vi "AMS Gas v2.0.vi"() -> ()   [LabVIEW 2015]
uses:
  Controls/FP Sample Container.ctl
  Controls/Valve Vertical.ctl
  Controls/Valve Custom.ctl
  Controls/Freezer.ctl
  Controls/Scroll ONOFF.ctl
  Controls/Sample Transfer State Enumerator.ctl
  Controls/Sample Push State Enumerator.ctl
  Controls/Vacuum State Enumerator.ctl
  Controls/FP Control Refs Cluster.ctl
  Controls/Liquid N Valve Ref Cluster.ctl
  Controls/Main Line Valve Ref Cluster.ctl
  Controls/Sample Valve Refs.ctl
  Controls/Syringe Ctrl Refs.ctl
  Controls/AMS Gas State Enumerator.ctl
  AMS Gas/AMS Gas.lvclass
  <vilib>/ActorFramework/Message Enqueuer/Message Enqueuer.lvclass/Message Enqueuer.ctl
  Controls/Sample Line State Enumerator.ctl
  Controls/Sample Transfer Control Enumerator.ctl
  Controls/Sample Push Control Enumerator.ctl
  <vilib>/ActorFramework/Message Enqueuer/Enqueue.vi
  <vilib>/ActorFramework/Message Priority Queue/Priority Enqueue.vi
  AMS Gas Messages/Open Log Msg/Open Log Msg.lvclass
  AMS Gas Messages/Open Thermocouples Msg/Open Thermocouples Msg.lvclass
  <vilib>/ActorFramework/Stop Msg/Stop Msg.lvclass
panel:
  out "Syringe TC 2":dbl(slide)
  out "Sample Transfer State":T1
  out "Sample Push Progress Slide":u8(slide) scale=0.0..100.0
  in  "Syringe TC Graph":bool
  out "Sample Push State":T2
  out "Syringe TC":dbl(slide) scale=-200.0..50.0
  in  "Open Log":bool
  in  "Blank Button":bool
  out "Vacuum State":T3=enum."Unknown"
  out "Baratron 1":dbl(knob) scale=0.0005..1000.0
  in  "Vacuum Derivative":dbl(slide) scale=-0.01..0.01
  in  "Cylinder Home":bool
  in  "Syringe Blower":bool
  in  "Syringe Freeze":bool
  in  "Syringe Heater":bool
  in  "Piston Heater":bool
  in  "Syringe Valve":bool
  in  "Capillary Valve":bool
  in  "Syringe Container":bool
  out "Sample Transfer Progress Slide":u8(slide) scale=0.0..100.0
  in  "Cylinder Setpoint":dbl=2.6 min=0.0 max=10.0 step=0.01 format="%_3f bar"
  in  "He Line Valve DV318":bool
  in  "Push Time (sec)":dbl=inf
  out "cRIO CPU":u8(slide) scale=0.0..100.0
  out "Capillary Container":bool
  in  "Monkey Mode":bool
  out "error out":errorcluster
  in  "Scroll ON/OFF":T4
  in  "Turbo ON":bool
  out "Turbo Speed":dbl(knob) scale=0.0..100.0
  in  "Turbo Valve DV313":bool
  in  "Turbo Line Container":T5
  in  "GV400":T6
  in  "GV401":T6
  out "FV Gauge":dbl
  out "Log":string
  in  "Liquid N Master Valve HV 107":bool
  in  "Cold Bath Syringe HV 106":bool
  in  "Cold Bath Storage 1 HV 102":T7
  in  "Cold Bath Storage 2 HV 103":T7
  in  "Cold Bath Storage 3 HV 104":bool
  in  "Cold Bath Storage 4 HV 105":bool
  in  "Tank Blower 4":bool
  in  "Tank Blower 3":bool
  in  "Tank Blower 2":bool
  in  "Tank Blower 1":bool
  in  "Clear Charts":bool
  out "Baratrons Chart":cluster{"mean":dbl, "mean":dbl}(graph)
  out "Baratron 1":dbl(knob) scale=0.5..1000.0
  in  "Storage Valve 1":bool
  in  "Storage Valve 2":bool
  in  "Storage Valve 3":bool
  in  "Storage Valve 4":bool
  in  "Storage Valve 5":bool
  in  "Storage Valve 6":bool
  in  "Storage Valve 7":bool
  in  "Storage Valve 9":bool
  in  "Storage Valve 0":bool
  in  "Storage Valve 11":bool
  in  "Storage Valve 12":bool
  in  "Storage Valve 8":bool
  in  "Storage Container 1":T5
  in  "Storage Container 2":T5
  in  "Storage Container 3":T5
  in  "Storage Container 4":T5
  in  "Storage Container 5":T5
  in  "Storage Container 6":T5
  in  "Storage Container 7":T5
  in  "Storage Container 8":T5
  in  "Storage Container 9":T5
  in  "Storage Container 10":T5
  in  "Storage Container 11":T5
  in  "Storage Container 12":T5
  in  "Prep Line Valve 0 DV300":bool
  in  "Sample 1 DV314":bool
  in  "Sample 2 DV315":bool
  in  "Sample 3 DV316":bool
  in  "Sample 4 DV317":bool
  in  "Sample 5 DV318":bool
  in  "Sample 1":bool
  in  "Sample 2":bool
  in  "Sample 3":bool
  in  "Sample 4":bool
  in  "Sample 5":bool
  in  "Transfer Line Container":bool=TRUE
  in  "Preparation Container":bool
  in  "Cold Bath 1 Freeze":T8
  in  "Cold Bath 2 Freeze":T8
  in  "Cold Bath 3 Freeze":T8
  in  "Cold Bath 4 Freeze":T8
  in  "Cylinder Container":bool
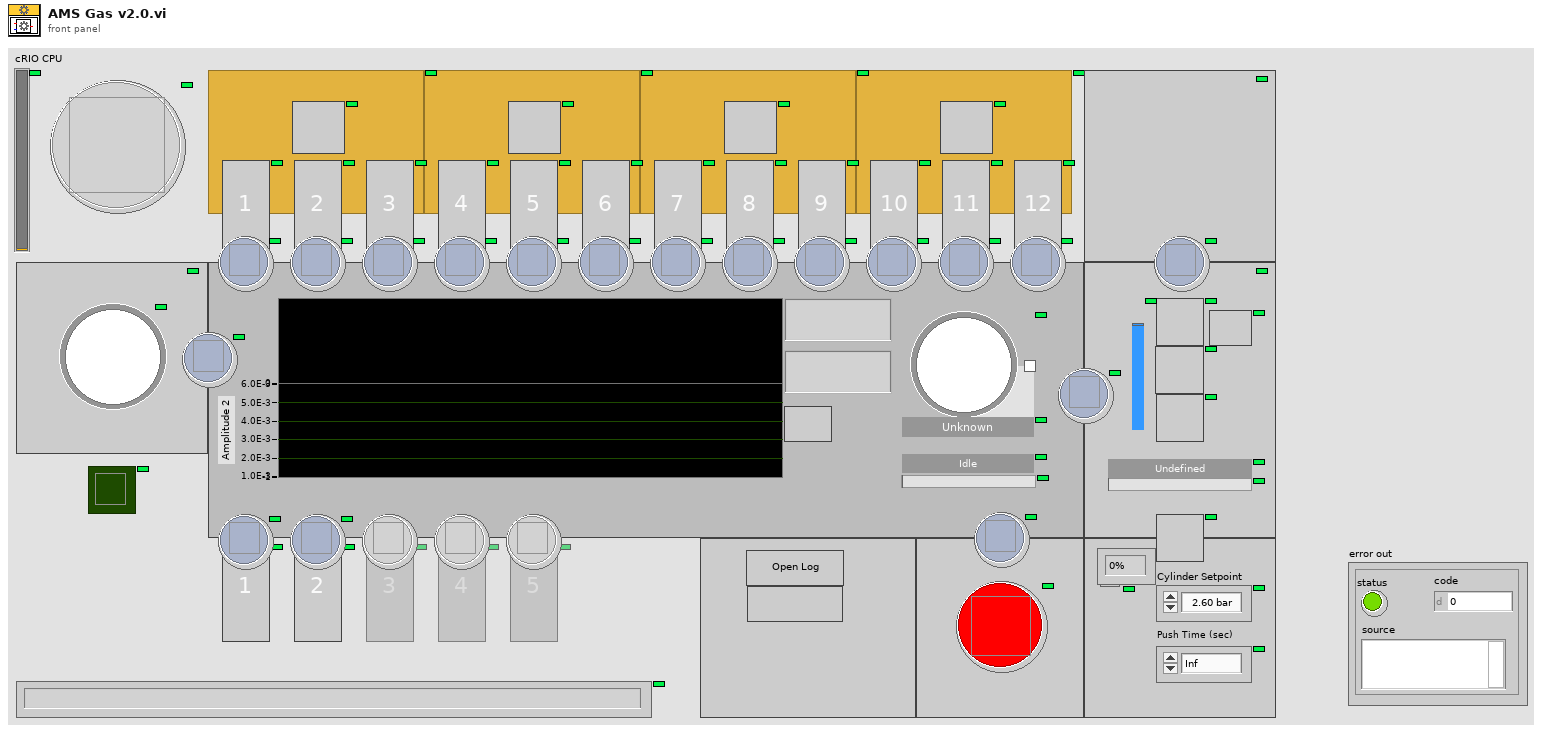
[diagram p1: front panel]
types:
  T1 = typedef "Sample Transfer State Enumerator.ctl" = enum16{"Idle", "Initialize", "Check Containers", "Check Temperatures", "Start Turbo", "Warm Up Containers", "Prepare for purging", "Purge Capillary", "Purge", "Open Containers", "Introduce Sample", "Measure Base Pressure", "Home Syringe", "Start Freezer", "Freeze Target", "Crystalize", "Initiate Stash", "Stash", "Polish", "Stop Freezers", "Push Sample", "Complete", "Abort", "Error", "Undefined"}
  T2 = typedef "Sample Push State Enumerator.ctl" = enum16{"Undefined", "Initialize", "Dilute", "Close Transfer Line", "Start Heaters", "Warm Up Syringe", "Ready to Push", "Push", "Initiate Stash", "Stash", "Complete", "Abort", "Idle", "Error"}
  T3 = typedef "Vacuum State Enumerator.ctl" = enum16{"Pressure Rising", "Plateau", "Pressure Dropping", "Valley", "Low Valley", "Leak", "Unknown"}
  T4 = typedef "Scroll ONOFF.ctl" = bool
  T5 = typedef "FP Sample Container.ctl" = bool
  T6 = typedef "Valve Vertical.ctl" = bool
  T7 = typedef "Valve Custom.ctl" = bool
  T8 = typedef "Freezer.ctl" = bool
  T9 = typedef "AMS Gas State Enumerator.ctl" = enum16{"Initialize", "Idle", "Change to Manual", "Change to Auto", "Shutdown"}
  T10 = typedef "FP Control Refs Cluster.ctl" = cluster{"Liquid N Valve References":T11, "Main Line Valve Refs":T12, "Transfer Line Container":refnum<vi>, "Storage Containers":refnum<vi>[], "Sample Refs":T13, "Syringe Ctrl Refs ":T14, "Baratrons Chart":refnum<vi>, "Capillary Container":refnum<vi>, "Preparation Container":refnum<vi>, "Monkey Mode":refnum<vi>}
  T11 = typedef "Liquid N Valve Ref Cluster.ctl" = cluster{"Cold Bath H2O HV 100":refnum<vi>, "Cold Bath Cleaning HV 101":refnum<vi>, "Cold Bath Storage 1 HV 102":refnum<vi>, "Cold Bath Storage 2 HV 103":refnum<vi>, "Cold Bath Storage 3 HV 104":refnum<vi>, "Cold Bath Storage 4 HV 105":refnum<vi>, "Cold Bath Syringe HV 106":refnum<vi>, "Liquid N Master Valve HV 107":refnum<vi>}
  T12 = typedef "Main Line Valve Ref Cluster.ctl" = cluster{"Turbo Valve DV313":refnum<vi>, "Prep Line Valve 0 DV300":refnum<vi>, "Storage Valves":refnum<vi>[]}
  T13 = typedef "Sample Valve Refs.ctl" = cluster{"Valves":cluster{"Sample 5 DV318":refnum<vi>, "Sample 4 DV317":refnum<vi>, "Sample 3 DV316":refnum<vi>, "Sample 2 DV315":refnum<vi>, "Sample 1 DV314":refnum<vi>}, "Lines":cluster{"Sample 1":refnum<vi>, "Sample 2":refnum<vi>, "Sample 3":refnum<vi>, "Sample 4":refnum<vi>, "Sample 5":refnum<vi>}}
  T14 = typedef "Syringe Ctrl Refs.ctl" = cluster{"Syringe Home":refnum<vi>, "Syringe Freeze":refnum<vi>, "Syringe TC":refnum<vi>, "Syringe Container":refnum<vi>}
  T15 = typedef "Sample Line State Enumerator.ctl" = enum16{"All lines closed", "Sample line 1.", "Sample line 2.", "Sample line 3.", "Sample line 4.", "Sample line 5.", "Out of range"}
  T16 = typedef "Sample Transfer Control Enumerator.ctl" = enum16{"Acknowledged", "Transfer", "Stash", "Abort", "Reset to Idle"}
  T17 = typedef "Sample Push Control Enumerator.ctl" = enum16{"Acknowledged", "Push", "Stash", "Abort", "Reset to Idle"}
  T18 = typedef "Sample Container.ctl" = cluster{"Sample In":refnum<k21>, "Sample Name":refnum<k21>, "Ti Cathode":refnum<k21>, "SampleQ":refnum<queue>}
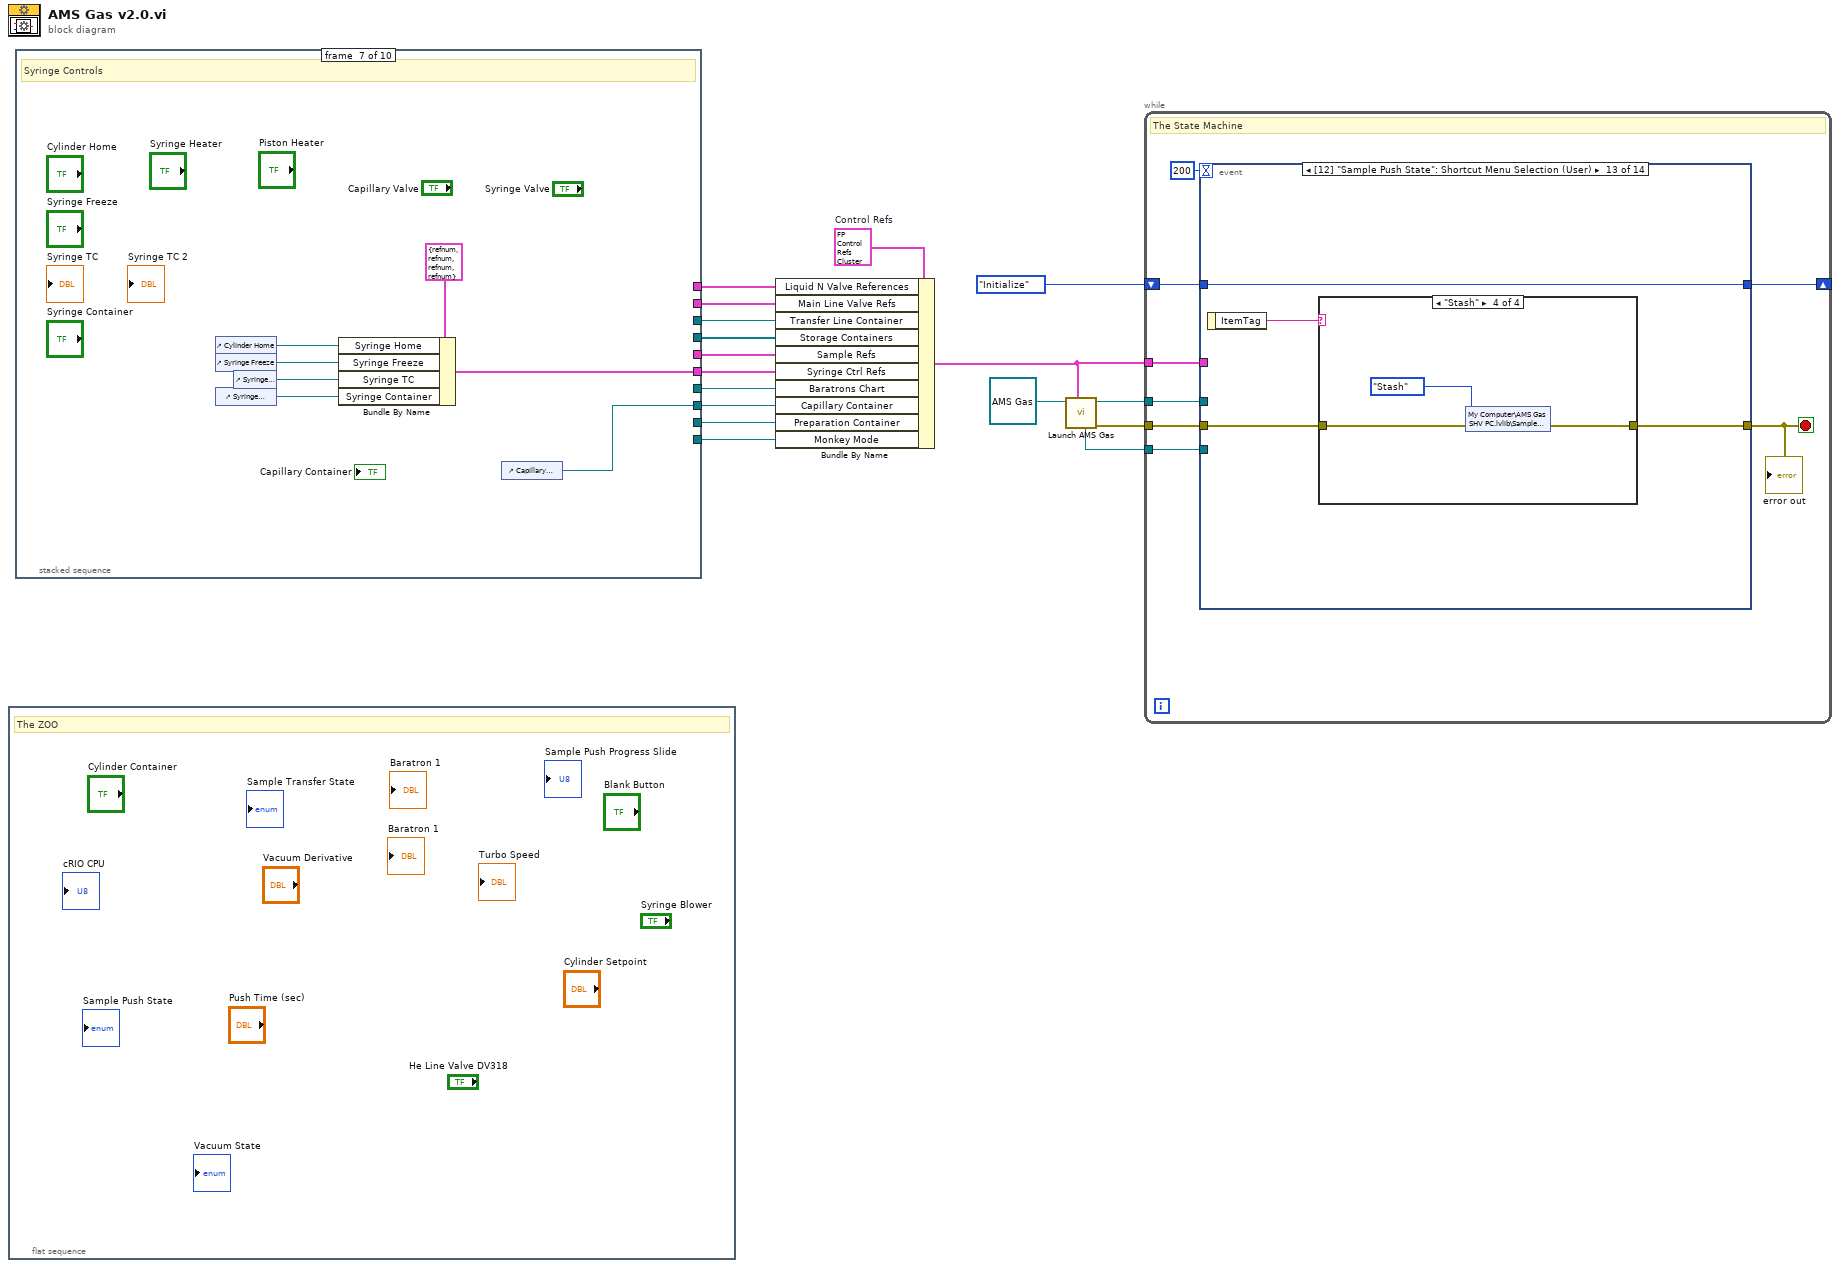
[diagram p0: block diagram]
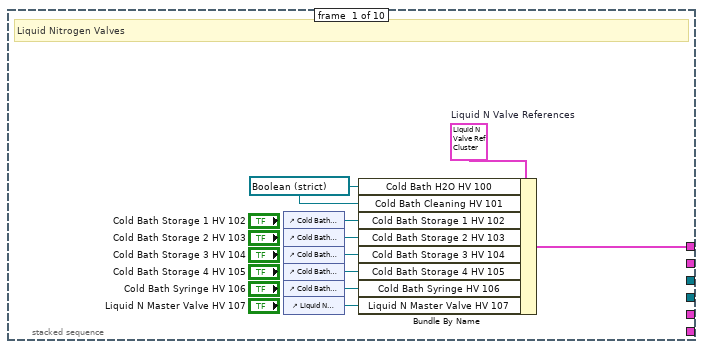
[diagram p2: hidden frame]
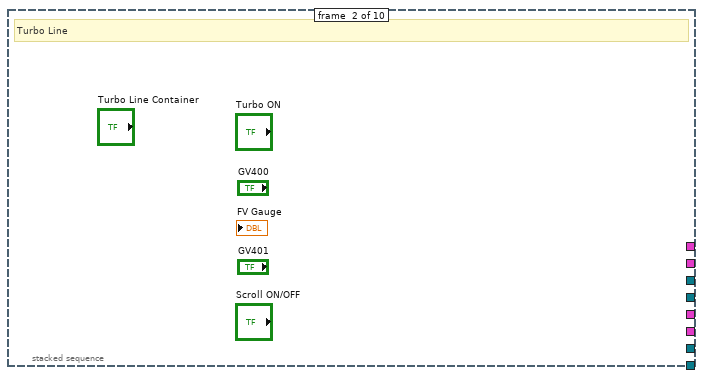
[diagram p3: hidden frame]
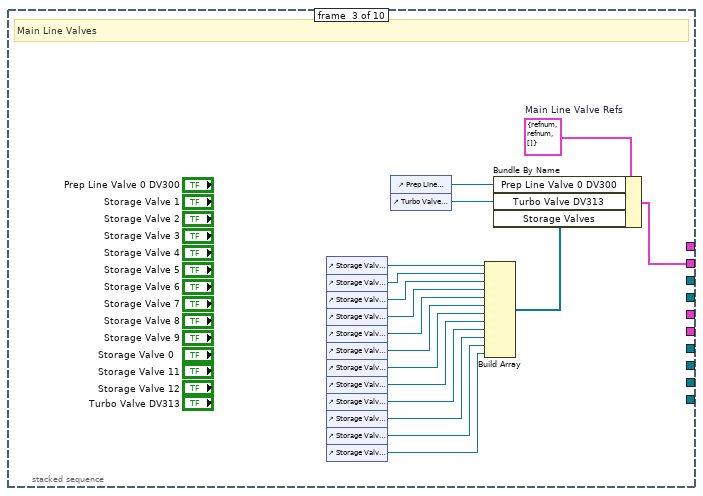
[diagram p4: hidden frame]
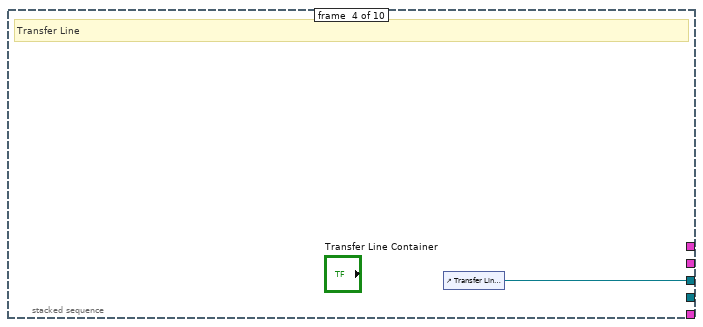
[diagram p5: hidden frame]
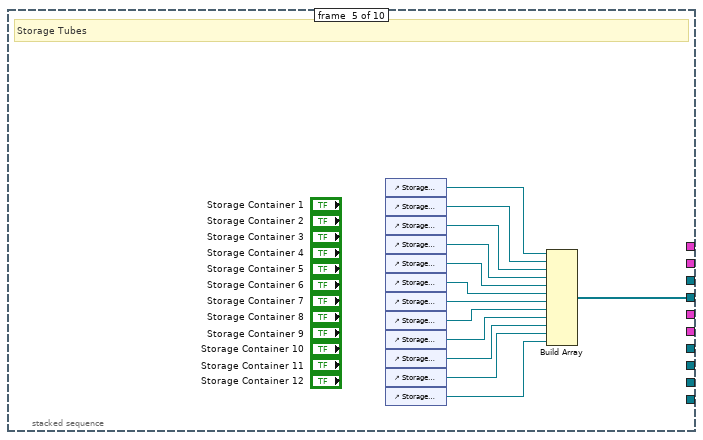
[diagram p6: hidden frame]
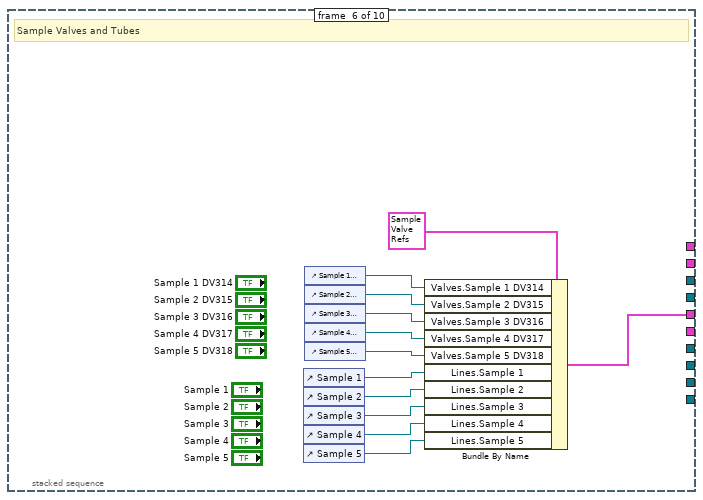
[diagram p7: hidden frame]
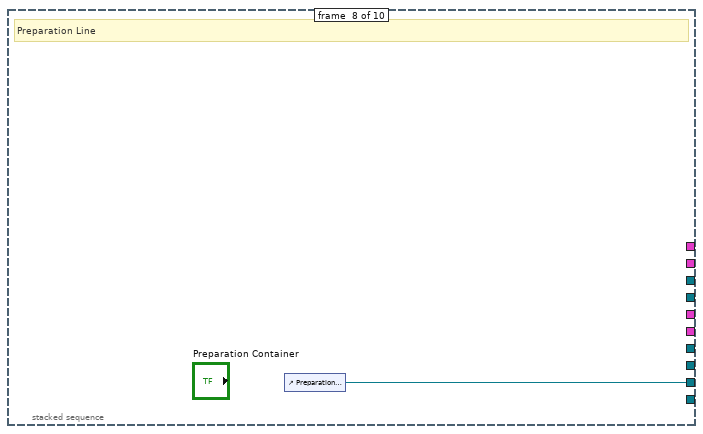
[diagram p8: hidden frame]
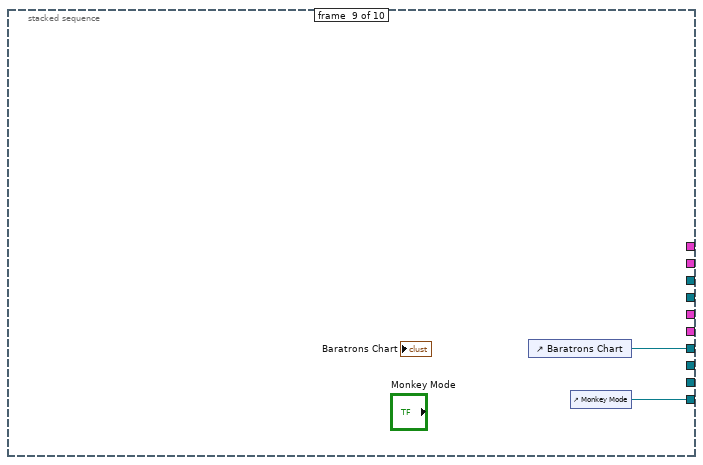
[diagram p9: hidden frame]
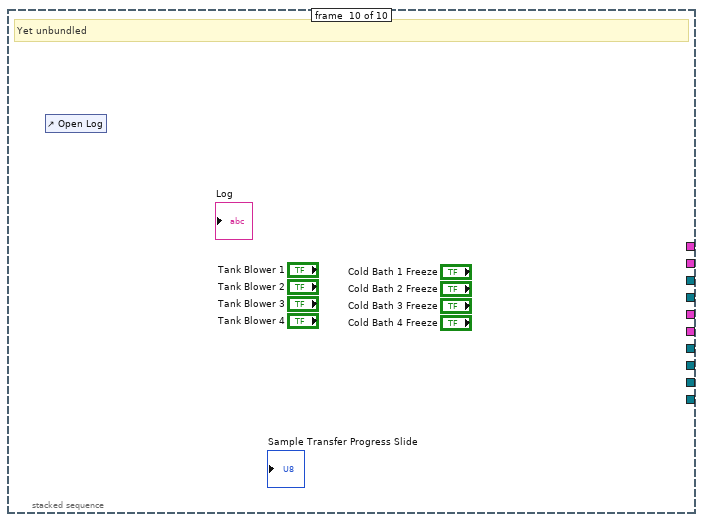
[diagram p10: hidden frame]
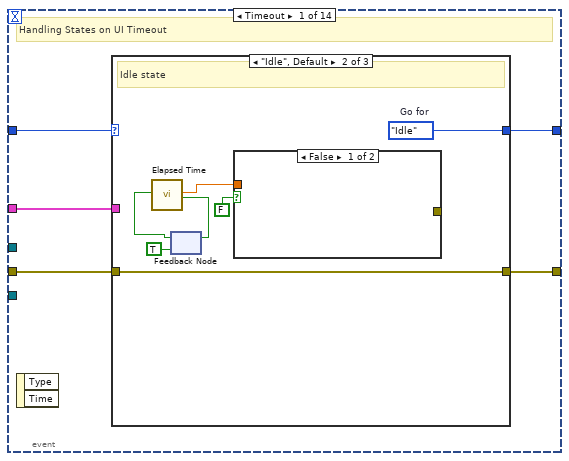
[diagram p11: hidden frame]
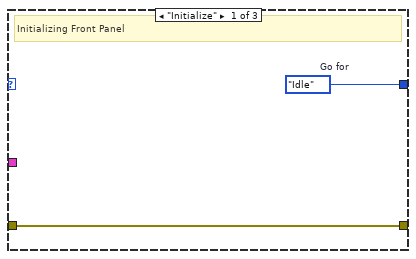
[diagram p12: hidden frame]
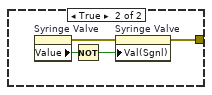
[diagram p13: hidden frame]
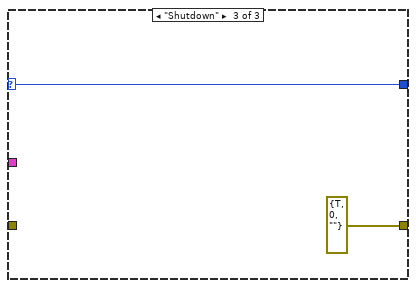
[diagram p14: hidden frame]
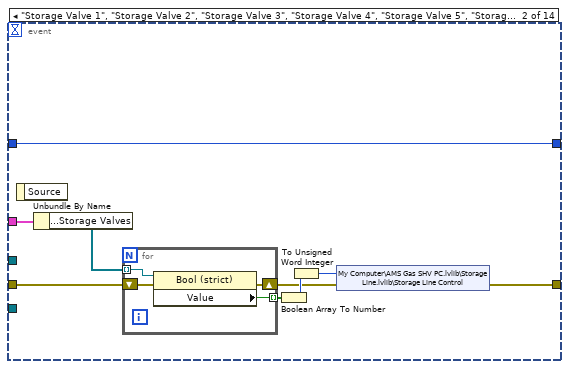
[diagram p15: hidden frame]
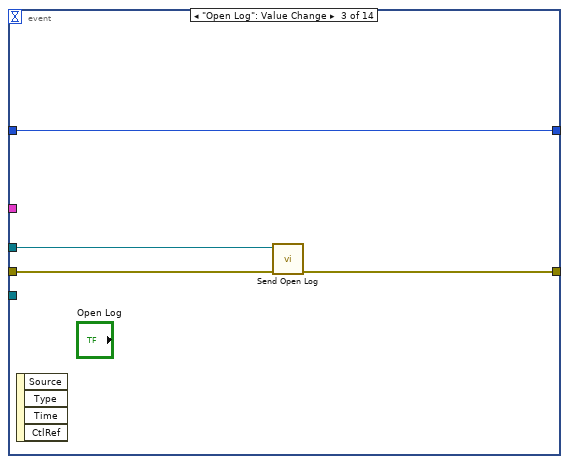
[diagram p16: hidden frame]
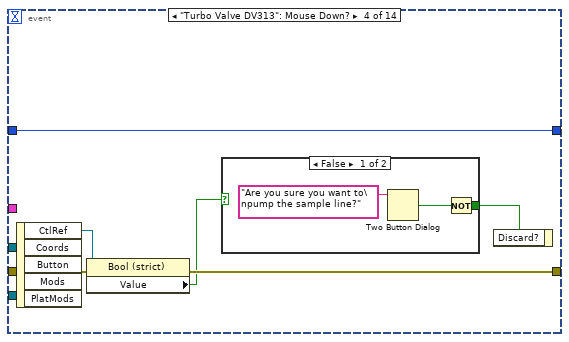
[diagram p17: hidden frame]
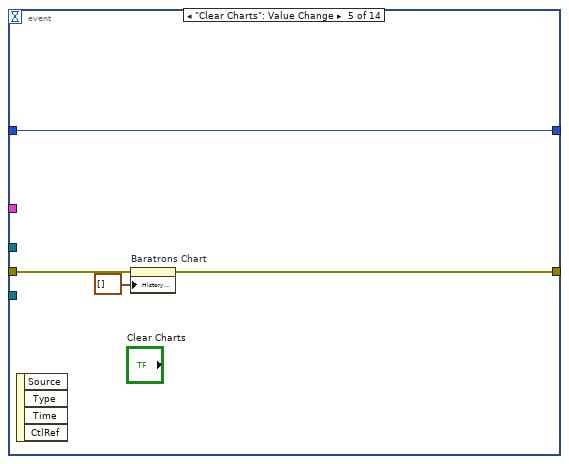
[diagram p19: hidden frame]
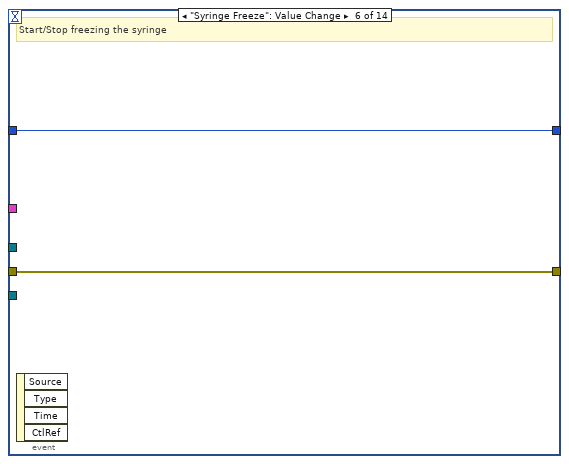
[diagram p20: hidden frame]
diagram:
  w17 = T10 {"Liquid N Valve References"={"Cold Bath H2O HV 100"=refnum, "Cold Bath Cleaning HV 101"=refnum, "Cold Bath Storage 1 HV 102"=refnum, "Cold Bath Storage 2 HV 103"=refnum, "Cold Bath Storage 3 HV 104"=refnum, "Cold Bath Storage 4 HV 105"=refnum, "Cold Bath Syringe HV 106"=refnum, "Liquid N Master Valve HV 107"=refnum}, "Main Line Valve Refs"={"Turbo Valve DV313"=refnum, "Prep Line Valve 0 DV300"=refnum, "Storage Valves"=[]}, "Transfer Line Container"=refnum, "Storage Containers"=[], "Sample Refs"={"Valves"={"Sample 5 DV318"=refnum, "Sample 4 DV317"=refnum, "Sample 3 DV316"=refnum, "Sample 2 DV315"=refnum, "Sample 1 DV314"=refnum}, "Lines"={"Sample 1"=refnum, "Sample 2"=refnum, "Sample 3"=refnum, "Sample 4"=refnum, "Sample 5"=refnum}}, "Syringe Ctrl Refs "={"Syringe Home"=refnum, "Syringe Freeze"=refnum, "Syringe TC"=refnum, "Syringe Container"=refnum}, "Baratrons Chart"=refnum, "Capillary Container"=refnum, "Preparation Container"=refnum, "Monkey Mode"=refnum}  # Control Refs
  n1 = flat-sequence {
    frame #0 {
      # "The ZOO"
    }
  }
  n2 = stacked-sequence {
    tunnel: [_ _ w43 _ _ _ _ _ _ _] -> w16
    tunnel: [_ _ _ _ w45 _ _ _ _ _] -> w13
    tunnel: [_ _ _ _ _ w63 _ _ _ _] -> w12
    tunnel: [w19 _ _ _ _ _ _ _ _ _] -> w14
    tunnel: [_ _ _ _ _ _ w75 _ _ _] -> w11
    tunnel: [_ _ _ _ _ _ _ _ w79 _] -> w8
    tunnel: [_ _ _ _ _ _ w71 _ _ _] -> w6
    tunnel: [_ _ _ _ _ _ _ w77 _ _] -> w5
    tunnel: [_ _ _ w44 _ _ _ _ _ _] -> w3
    tunnel: [_ _ _ _ _ _ _ _ w78 _] -> w1
    frame #0 {
      w18 = refnum<vi> refnum ("Cold Bath H2O HV 100")
      w26 = T11 {"Cold Bath H2O HV 100"=refnum, "Cold Bath Cleaning HV 101"=refnum, "Cold Bath Storage 1 HV 102"=refnum, "Cold Bath Storage 2 HV 103"=refnum, "Cold Bath Storage 3 HV 104"=refnum, "Cold Bath Storage 4 HV 105"=refnum, "Cold Bath Syringe HV 106"=refnum, "Liquid N Master Valve HV 107"=refnum}  # Liquid N Valve References
      # "Liquid Nitrogen Valves"
      n3 = control-ref of="Cold Bath Storage 1 HV 102"() -> (w20:refnum<vi>)
      n4 = control-ref of="Cold Bath Storage 2 HV 103"() -> (w21:refnum<vi>)
      n5 = control-ref of="Cold Bath Storage 3 HV 104"() -> (w22:refnum<vi>)
      n6 = control-ref of="Cold Bath Storage 4 HV 105"() -> (w23:refnum<vi>)
      n7 = control-ref of="Cold Bath Syringe HV 106"() -> (w24:refnum<vi>)
      n8 = control-ref of="Liquid N Master Valve HV 107"() -> (w25:refnum<vi>)
      n9 = Bundle By Name(cluster=w26, "Cold Bath H2O HV 100"=w18, "Cold Bath Cleaning HV 101"=w18, "Cold Bath Storage 1 HV 102"=w20, "Cold Bath Storage 2 HV 103"=w21, "Cold Bath Storage 3 HV 104"=w22, "Cold Bath Storage 4 HV 105"=w23, "Cold Bath Syringe HV 106"=w24, "Liquid N Master Valve HV 107"=w25) -> (w19:T11)
    }
    frame #1 {
      # "Turbo Line"
    }
    frame #2 {
      w42 = T12 {"Turbo Valve DV313"=refnum, "Prep Line Valve 0 DV300"=refnum, "Storage Valves"=[]}  # Main Line Valve Refs
      # "Main Line Valves"
      n10 = control-ref of="Storage Valve 1"() -> (w41:refnum<vi>)
      n11 = control-ref of="Storage Valve 2"() -> (w40:refnum<vi>)
      n12 = control-ref of="Storage Valve 3"() -> (w39:refnum<vi>)
      n13 = control-ref of="Storage Valve 4"() -> (w38:refnum<vi>)
      n14 = control-ref of="Storage Valve 5"() -> (w37:refnum<vi>)
      n15 = control-ref of="Storage Valve 6"() -> (w36:refnum<vi>)
      n16 = control-ref of="Storage Valve 7"() -> (w35:refnum<vi>)
      n17 = control-ref of="Storage Valve 8"() -> (w34:refnum<vi>)
      n18 = control-ref of="Storage Valve 9"() -> (w33:refnum<vi>)
      n19 = control-ref of="Storage Valve 0"() -> (w32:refnum<vi>)
      n20 = control-ref of="Storage Valve 11"() -> (w31:refnum<vi>)
      n21 = control-ref of="Storage Valve 12"() -> (w30:refnum<vi>)
      n22 = control-ref of="Prep Line Valve 0 DV300"() -> (w28:refnum<vi>)
      n23 = control-ref of="Turbo Valve DV313"() -> (w27:refnum<vi>)
      n24 = Build Array(w41, w40, w39, w38, w37, w36, w35, w34, w33, w32, w31, w30) -> (w29:refnum<vi>[])
      n25 = Bundle By Name(cluster=w42, "Prep Line Valve 0 DV300"=w28, "Turbo Valve DV313"=w27, "Storage Valves"=w29) -> (w43:T12)
    }
    frame #3 {
      # "Transfer Line"
      n26 = control-ref of="Transfer Line Container"() -> (w44:refnum<vi>)
    }
    frame #4 {
      # "Storage Tubes"
      n27 = control-ref of="Storage Container 1"() -> (w50:refnum<vi>)
      n28 = control-ref of="Storage Container 2"() -> (w51:refnum<vi>)
      n29 = control-ref of="Storage Container 3"() -> (w54:refnum<vi>)
      n30 = control-ref of="Storage Container 4"() -> (w53:refnum<vi>)
      n31 = control-ref of="Storage Container 5"() -> (w52:refnum<vi>)
      n32 = control-ref of="Storage Container 6"() -> (w48:refnum<vi>)
      n33 = control-ref of="Storage Container 7"() -> (w55:refnum<vi>)
      n34 = control-ref of="Storage Container 8"() -> (w47:refnum<vi>)
      n35 = control-ref of="Storage Container 9"() -> (w49:refnum<vi>)
      n36 = control-ref of="Storage Container 10"() -> (w56:refnum<vi>)
      n37 = control-ref of="Storage Container 11"() -> (w57:refnum<vi>)
      n38 = control-ref of="Storage Container 12"() -> (w46:refnum<vi>)
      n39 = Build Array(w50, w51, w54, w53, w52, w48, w55, w47, w49, w56, w57, w46) -> (w45:refnum<vi>[])
    }
    frame #5 {
      # "Sample Valves and Tubes"
      n40 = control-ref of="Sample 1"() -> (w62:refnum<vi>)
      n41 = control-ref of="Sample 2"() -> (w61:refnum<vi>)
      n42 = control-ref of="Sample 3"() -> (w60:refnum<vi>)
      n43 = control-ref of="Sample 4"() -> (w59:refnum<vi>)
      n44 = control-ref of="Sample 5"() -> (w58:refnum<vi>)
      n45 = control-ref of="Sample 1 DV314"() -> (w69:refnum<vi>)
      n46 = control-ref of="Sample 2 DV315"() -> (w68:refnum<vi>)
      n47 = control-ref of="Sample 3 DV316"() -> (w67:refnum<vi>)
      n48 = control-ref of="Sample 4 DV317"() -> (w66:refnum<vi>)
      n49 = control-ref of="Sample 5 DV318"() -> (w65:refnum<vi>)
      n50 = Bundle By Name(cluster=T13 {"Valves"={"Sample 5 DV318"=refnum, "Sample 4 DV317"=refnum, "Sample 3 DV316"=refnum, "Sample 2 DV315"=refnum, "Sample 1 DV314"=refnum}, "Lines"={"Sample 1"=refnum, "Sample 2"=refnum, "Sample 3"=refnum, "Sample 4"=refnum, "Sample 5"=refnum}} ("Sample Valve Refs"), "Valves.Sample 1 DV314"=w69, "Valves.Sample 2 DV315"=w68, "Valves.Sample 3 DV316"=w67, "Valves.Sample 4 DV317"=w66, "Valves.Sample 5 DV318"=w65, "Lines.Sample 1"=w62, "Lines.Sample 2"=w61, "Lines.Sample 3"=w60, "Lines.Sample 4"=w59, "Lines.Sample 5"=w58) -> (w63:T13)
    }
    frame #6 {
      # "Syringe Controls"
      n51 = control-ref of="Cylinder Home"() -> (w72:refnum<vi>)
      n52 = control-ref of="Syringe Freeze"() -> (w74:refnum<vi>)
      n53 = control-ref of="Syringe Container"() -> (w70:refnum<vi>)
      n54 = control-ref of="Syringe TC"() -> (w73:refnum<vi>)
      n55 = Bundle By Name(cluster=T14 {"Syringe Home"=refnum, "Syringe Freeze"=refnum, "Syringe TC"=refnum, "Syringe Container"=refnum} ("Syringe Ctrl Refs"), "Syringe Home"=w72, "Syringe Freeze"=w74, "Syringe TC"=w73, "Syringe Container"=w70) -> (w75:T14)
      n56 = control-ref of="Capillary Container"() -> (w71:refnum<vi>)
    }
    frame #7 {
      # "Preparation Line"
      n57 = control-ref of="Preparation Container"() -> (w77:refnum<vi>)
    }
    frame #8 {
      n58 = control-ref of="Baratrons Chart"() -> (w79:refnum<vi>)
      n59 = control-ref of="Monkey Mode"() -> (w78:refnum<vi>)
    }
    frame #9 {
      # "Yet unbundled"
      n60 = control-ref of="Open Log"() -> ()  [unwired: 1 out]
    }
  }
  n61 = Bundle By Name(cluster=w17, "Liquid N Valve References"=w14, "Main Line Valve Refs"=w16, "Transfer Line Container"=w3, "Storage Containers"=w13, "Sample Refs"=w12, "Syringe Ctrl Refs"=w11, "Baratrons Chart"=w8, "Capillary Container"=w6, "Preparation Container"=w5, "Monkey Mode"=w1) -> (w4:T10)
  n62 = call "Launch AMS Gas.vi"("Control Refs"=w4, "AMS Gas in"=refnum<class "AMS Gas.lvclass"> refnum) -> ("error out"=w7:errorcluster, "Caller-To-Actor Enqueuer"=w10:refnum<class "Message Enqueuer.lvclass">, "Sample Clipboard Q"=w2:refnum<queue>)  [unwired: 7 in]
  n63 = while {
    tunnel: w4 -> [w82]
    tunnel: w7 -> [w87]
    shift-right: [w83] -> _
    shift-left: AMS_Gas_State_Enumerator."Initialize" ("Go for") -> [w84]
    tunnel: w10 -> [w81]
    tunnel: w2 -> [w80]
    stop <- w86 stop-if-true
    # "The State Machine"
    n64 = event shown="[12] \"Sample Push State\": Shortcut Menu Selection (User)" {
      selector: _ -> [_ _ _ _ _ _ _ _ _ _ _ _ _ _]
      dyn-events: _ -> [_ _ _ _ _ _ _ _ _ _ _ _ _ _]
      timeout: 200 -> [_ _ _ _ _ _ _ _ _ _ _ _ _ _]
      tunnel: w87 -> [w92 w114 w123 w129 w137 w138 w140 w144 w148 w161 w170 w175 w191 w208]
      tunnel: [w91 w109 w122 w128 w134 w138 w140 w142 w147 w151 w171 w173 w189 w207] -> w86
      tunnel: w84 -> [w90 w116 w124 w130 w136 w139 w141 w145 _ w162 w172 w176 w192 w209]
      tunnel: [w89 w116 w124 w130 w136 w139 w141 w145 w150 w162 w172 w176 w192 w209] -> w83
      tunnel: w82 -> [w88 w115 _ _ _ _ _ _ _ _ _ _ _ w206]
      tunnel: w81 -> [_ _ w121 _ _ _ _ w143 w146 _ _ _ _ _]
      tunnel: w80 -> [_ _ _ _ _ _ _ _ _ _ w168 _ _ _]
      event Timeout {
        # "Handling States on UI Timeout"
        n65 = event-data() -> ()  [unwired: 1 in, 2 out]
        n66 = case shown="\"Idle\", Default" w90 {
          selector: w90 -> [_ _ w107]
          tunnel: w92 -> [w93 w100 _]
          tunnel: [w93 w100 errorcluster {"status"=TRUE, "code"=0, "source"=""} ("no error")] -> w91
          tunnel: [w94 w101 w107] -> w89
          tunnel: w88 -> [_ _ _]
          frame "Initialize" {
            w94 = AMS_Gas_State_Enumerator."Idle"  # Go for
            # "Initializing Front Panel"
          }
          frame "Idle", Default {
            w101 = AMS_Gas_State_Enumerator."Idle"  # Go for
            # "Idle state"
            n67 = feedback #1(TRUE ("Time has Elapsed")) -> (w99:bool)
            n68 = call "Elapsed Time"("Reset"=w99) -> ("Elapsed Time (s)"=w97:dbl, "Time has Elapsed"=w96:bool)  [unwired: 11 in, 6 out]
            n69 = feedback-in #1(w96) -> ()
            n70 = case shown="False" FALSE {
              tunnel: [_ w102] -> _
              tunnel: w97 -> [_ _]
              frame False {
              }
              frame True {
                n71 = property on="Syringe Valve" class="Bool (strict)"() -> (error out=w103:errorcluster, "Value"=w105:bool)  [unwired: 2 in, 1 out]
                n72 = Not(x=w105) -> (.not. x?=w104:bool)
                n73 = property on="Syringe Valve" class="Bool (strict)"(error in=w103, "Val(Sgnl)"=w104) -> (error out=w102:errorcluster)  [unwired: 1 in, 1 out]
              }
            }
          }
          frame "Shutdown" {
          }
        }
      }
      event "Storage Valve 1", "Storage Valve 2", "Storage Valve 3", "Storage Valve 4", "Storage Valve 5", "Storage Valve 6", "Storage Valve 7", "Storage Valve 9", "Storage Valve 0", "Storage Valve 11", "Storage Valve 12", "Storage Valve 8": Value Change {
        n74 = event-data() -> ()  [unwired: 1 in, 1 out]
        n75 = Unbundle By Name(w115) -> ("Main Line Valve Refs.Storage Valves"=w108:refnum<vi>[])
        n76 = for {
          tunnel: w108 -> [w118] mode=indexing
          tunnel: [w117] -> w113 mode=indexing
          shift-right: [w119] -> w111
          shift-left: w114 -> [w120]
          n77 = property class="Bool (strict)"(reference=w118, error in=w120) -> (error out=w119:errorcluster, "Value"=w117:bool)  [unwired: 1 out]
        }
        n78 = Boolean Array To Number(Boolean array=w113) -> (number=w112:u32)
        n79 = To Unsigned Word Integer(number=w112) -> (unsigned 16bit integer=w110:u16)
        n80 = shared-variable "My Computer\\AMS Gas SHV PC.lvlib\\Storage Line.lvlib\\Storage Line Control"(w110, error in=w111) -> (error out=w109:errorcluster)
      }
      event "Open Log": Value Change {
        n81 = event-data() -> ()  [unwired: 1 in, 4 out]
        n82 = call "Send Open Log.vi"("error in (no error)"=w123, "Message Enqueuer"=w121) -> ("error out"=w122:errorcluster)  [unwired: 8 in, 1 out]
      }
      event "Turbo Valve DV313": Mouse Down? {
        n83 = event-data() -> ("CtlRef"=w127:refnum<vi>)  [unwired: 1 in, 4 out]
        n84 = property class="Bool (strict)"(reference=w127, error in=w129) -> (error out=w128:errorcluster, "Value"=w126:bool)  [unwired: 1 out]
        n85 = case shown="False" w126 {
          tunnel: [w132 _] -> w125
          frame False {
            n86 = Two Button Dialog(message="Are you sure you want to\npump the sample line?") -> (T button?=w133:bool)  [unwired: 2 in]
            n87 = Not(x=w133) -> (.not. x?=w132:bool)
          }
          frame True {
          }
        }
        n88 = event-data("Discard?"=w125) -> ()  [unwired: 1 in, 1 out]
      }
      event "Clear Charts": Value Change {
        n89 = event-data() -> ()  [unwired: 1 in, 4 out]
        n90 = property on="Baratrons Chart" class="WFChart (strict)"(error in=w137, "History Data"=cluster{"mean":dbl, "mean":dbl}[] []) -> (error out=w134:errorcluster)  [unwired: 1 in, 1 out]
      }
      event "Syringe Freeze": Value Change {
        # "Start/Stop freezing the syringe"
        n91 = event-data() -> ()  [unwired: 1 in, 4 out]
      }
      event Value Change {
        # "Start/Stop freezing the Cold Bath 4"
        n92 = event-data() -> ()  [unwired: 1 in, 4 out]
      }
      event "Syringe TC Graph": Value Change {
        n93 = event-data() -> ()  [unwired: 1 in, 4 out]
        n94 = call "Send Open Thermocouples.vi"("error in (no error)"=w144, "Message Enqueuer"=w143) -> ("error out"=w142:errorcluster)  [unwired: 8 in, 1 out]
      }
      event Panel Close? {
        w150 = AMS_Gas_State_Enumerator."Shutdown"  # Go for
        # "User closes Front Panel"
        n95 = event-data() -> ()  [unwired: 1 in, 3 out]
        n96 = call <vilib>:"Send Normal Stop.vi"("error in (no error)"=w148, "Message Enqueuer"=w146) -> ("error out"=w147:errorcluster)  [unwired: 9 in]
        n97 = event-data("Discard?"=TRUE) -> ()  [unwired: 1 in, 1 out]
      }
      event "Sample 1 DV314", "Sample 2 DV315", "Sample 3 DV316", "Sample 4 DV317", "Sample 5 DV318": Mouse Down? {
        n98 = event-data() -> ("CtlRef"=w160:refnum<vi>)  [unwired: 1 in, 1 out]
        n99 = property class="Bool (strict)"(reference=w160, error in=w161) -> (error out=w152:errorcluster, "Label.Text"=w158:string, "Value"=w157:bool)  [unwired: 1 out]
        n100 = Not(x=w157) -> (.not. x?=w156:bool)
        n101 = case shown="\"Sample 2 DV315\"" w158 {
          tunnel: [Sample_Line_State_Enumerator."All lines closed" ("Sample Line") Sample_Line_State_Enumerator."Sample line 1." ("Sample Line") Sample_Line_State_Enumerator."Sample line 2." ("Sample Line")] -> w155
          frame "False", Default {
          }
          frame "Sample 1 DV314" {
          }
          frame "Sample 2 DV315" {
          }
        }
        n102 = Select(t=w155, s=w156, f=Sample_Line_State_Enumerator."All lines closed") -> (s? t:f=w153:T15)
        n103 = shared-variable "My Computer\\AMS Gas SHV PC.lvlib\\Sample Lines.lvlib\\Sample Line Control"(w153, error in=w152) -> (error out=w151:errorcluster)
        n104 = event-data("Discard?"=TRUE) -> ()  [unwired: 1 in, 1 out]
      }
      event "Syringe Container", "Transfer Line Container", "Preparation Container", "Sample 1", "Sample 2", "Capillary Container": Mouse Down {
        n105 = event-data() -> ("CtlRef"=w169:refnum<vi>)  [unwired: 1 in]
        n106 = call "Control to Sample Container.vi"("error in (no error)"=w170, "Sample Container Ref"=w169) -> ("error out"=w167:errorcluster, "Sample Container"=w166:T18)  [unwired: 8 in]
        n107 = call "Open Sample Container Dialog.vi"("error in (no error)"=w167, "Sample Clipboard Q"=w168, "Sample Container"=w166) -> ("error out"=w171:errorcluster)  [unwired: 8 in]
      }
      event Shortcut Menu Selection (User) {
        n108 = event-data() -> ("ItemTag"=w174:string)  [unwired: 1 in]
        n109 = case shown="\"Reset to Idle\"" w174 {
          selector: w174 -> [w178 _ _ _]
          tunnel: w175 -> [w179 w182 w185 w188]
          tunnel: [w179 w180 w183 w186] -> w173
          frame "False", Default {
            n110 = One Button Dialog(message=w178, button name ("OK")="Dismiss") -> ()  [unwired: 1 out]
          }
          frame "Reset to Idle" {
            n111 = shared-variable "My Computer\\AMS Gas SHV PC.lvlib\\Sample Transfer.lvlib\\Control"(Sample_Transfer_Control_Enumerator."Reset to Idle" ("Sample Transfer Control"), error in=w182) -> (error out=w180:errorcluster)
          }
          frame "Abort Transfer" {
            n112 = shared-variable "My Computer\\AMS Gas SHV PC.lvlib\\Sample Transfer.lvlib\\Control"(Sample_Transfer_Control_Enumerator."Abort" ("Sample Transfer Control"), error in=w185) -> (error out=w183:errorcluster)
          }
          frame "Stash" {
            n113 = shared-variable "My Computer\\AMS Gas SHV PC.lvlib\\Sample Transfer.lvlib\\Control"(Sample_Transfer_Control_Enumerator."Stash" ("Sample Transfer Control"), error in=w188) -> (error out=w186:errorcluster)
          }
        }
      }
      event Shortcut Menu Selection (User) {
        n114 = event-data() -> ("ItemTag"=w190:string)  [unwired: 1 in]
        n115 = case shown="\"Stash\"" w190 {
          selector: w190 -> [w194 _ _ _]
          tunnel: w191 -> [w195 w198 w201 w204]
          tunnel: [w195 w197 w200 w203] -> w189
          frame "False", Default {
            n116 = One Button Dialog(message=w194, button name ("OK")="Dismiss") -> ()  [unwired: 1 out]
          }
          frame "Reset to Idle" {
            n117 = shared-variable "My Computer\\AMS Gas SHV PC.lvlib\\Sample Push.lvlib\\Control"(Sample_Push_Control_Enumerator."Reset to Idle" ("Sample Push Control"), error in=w198) -> (error out=w197:errorcluster)
          }
          frame "Abort Push" {
            n118 = shared-variable "My Computer\\AMS Gas SHV PC.lvlib\\Sample Push.lvlib\\Control"(Sample_Push_Control_Enumerator."Abort" ("Sample Push Control"), error in=w201) -> (error out=w200:errorcluster)
          }
          frame "Stash" {
            n119 = shared-variable "My Computer\\AMS Gas SHV PC.lvlib\\Sample Push.lvlib\\Control"(Sample_Push_Control_Enumerator."Stash" ("Sample Push Control"), error in=w204) -> (error out=w203:errorcluster)
          }
        }
      }
      event "Monkey Mode": Value Change {
        n120 = event-data() -> ("NewVal"=w205:bool)  [unwired: 1 in]
        n121 = call "Set Monkey Mode.vi"("error in (no error)"=w208, "Monkey Mode"=w205, "Control Refs"=w206) -> ("error out"=w207:errorcluster)  [unwired: 8 in]
      }
    }
    "error out" <- w86
  }
